vi "Log Key Value Pairs.vi"(8 "error in (no error)":errorcluster, 9 "Numeric Array Key Value Pairs":cluster{"Key":string, "Value":dbl[]}[](array[cluster]), 10 "String Key Value Pairs":cluster{"Key":string, "Value":string}[](array[cluster]), 11 "SLL Spreadsheet Logger in":refnum<class "SLL CSV Logger.lvclass">) -> (0 "error out":errorcluster, 3 "SLL Spreadsheet Logger out":refnum<class "SLL CSV Logger.lvclass">)   [LabVIEW 2014, in "SLL Spreadsheet.lvlib" / "SLL CSV Logger.lvclass"]
doc: "Provide key-value pairs to be logged, where keys will be treated as Headers.\n\nFor numeric array key-value pairs provided, each value of the array will be logged as a new row in the file. The corresponding string key-value pairs will be duplicated for each of these rows."
uses:
  SLL CSV Logger.lvclass
  SLL CSV Logger.lvclass/SLL CSV Logger.ctl
  SLL Spreadsheet.lvlib
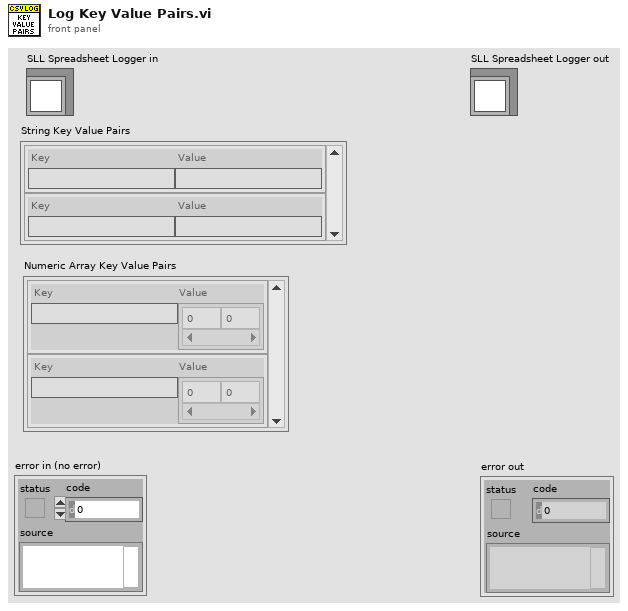
[diagram p1: front panel]
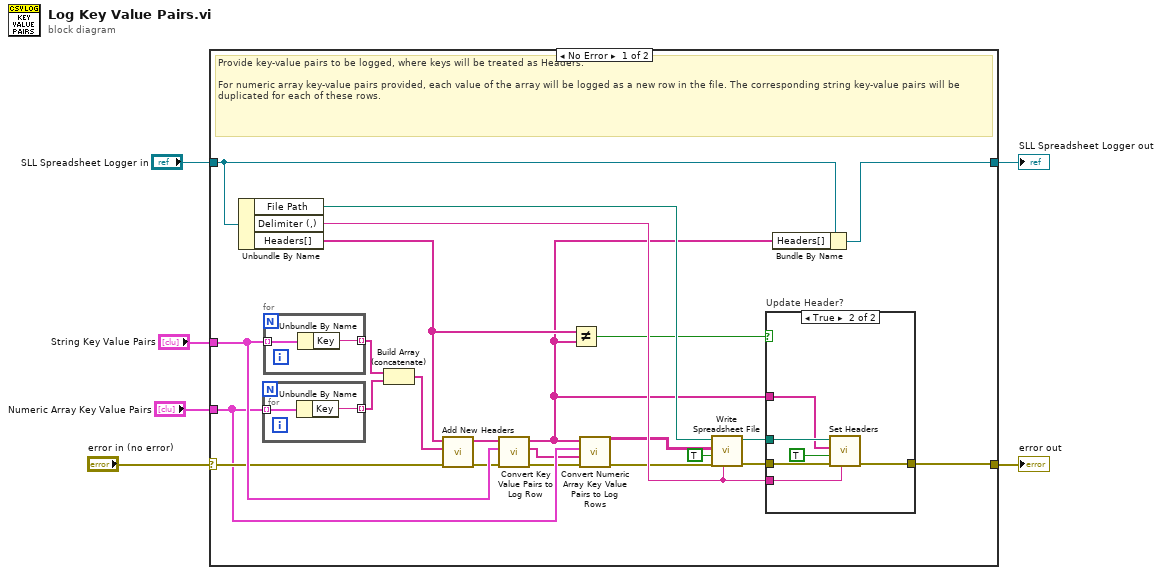
[diagram p0: block diagram]
diagram:
  n1 = case shown="No Error" "error in (no error)" {
    selector: "error in (no error)" -> [w16 w42]
    tunnel: [w21 w42] -> w5
    tunnel: [w28 w41] -> w3
    tunnel: "SLL Spreadsheet Logger in" -> [w29 w41]
    tunnel: "String Key Value Pairs" -> [w19 _]
    tunnel: "Numeric Array Key Value Pairs" -> [w11 _]
    frame No Error {
      # "Provide key-value pairs to be logged, where keys will be treated as Headers.\n\nFor numeric array key-value pairs provided, each value of the array will be logged as a new row in the file. The corresponding string key-value pairs will be duplicated for each of these rows."
      n2 = Unbundle By Name(w29) -> ("File Path"=w27:path, "Delimiter (,)"=w23:string, "Headers[]"=w20:string[])
      n3 = for {
        tunnel: w11 -> [w31] mode=indexing
        tunnel: [w30] -> w17 mode=indexing
        n4 = Unbundle By Name(w31) -> ("Key"=w30:string)
      }
      n5 = for {
        tunnel: w19 -> [w33] mode=indexing
        tunnel: [w32] -> w18 mode=indexing
        n6 = Unbundle By Name(w33) -> ("Key"=w32:string)
      }
      n7 = Build Array (concatenate)(w18, w17) -> (w15:string[])
      n8 = call "Add New Headers.vi"("error in (no error)"=w16, "Incoming Headers[]"=w15, "Existing Headers[]"=w20) -> ("error out"=w13:errorcluster, "Headers[] Out"=w14:string[])  [unwired: 7 in]
      n9 = call "Convert Key Value Pairs to Log Row.vi"("error in (no error)"=w13, "Key Value Pairs"=w19, "Headers In[]"=w14) -> ("error out"=w8:errorcluster, "Data Out[]"=w10:string[], "Headers Out[]"=w12:string[])  [unwired: 6 in]
      n10 = Not Equal?(x=w20, y=w12) -> (x != y?=w22:bool)
      n11 = call "Convert Numeric Array Key Value Pairs to Log Rows.vi"("error in (no error)"=w8, "Data[]"=w10, "Numeric Array Key Value Pairs"=w11, "Headers In[]"=w12) -> ("error out"=w7:errorcluster, "Log Data[][]"=w9:string[][])  [unwired: 6 in]
      n12 = call "Write Spreadsheet File.vi"("Delimiter (tab)"=w23, "error in (no error)"=w7, "Append to File? (F)"=TRUE, "2D String[][]"=w9, "File Path"=w27) -> ("error out"=w24:errorcluster, "File Path dup"=w25:path)  [unwired: 5 in]
      n13 = case "Update Header?" shown="True" w22 {
        tunnel: w25 -> [_ w40]
        tunnel: w24 -> [w34 w39]
        tunnel: w12 -> [_ w38]
        tunnel: w23 -> [_ w36]
        tunnel: [w34 w35] -> w21
        frame False {
        }
        frame True {
          n14 = call "Set Headers.vi"("Delimiter (,)"=w36, "error in (no error)"=w39, "Update Existing? (T)"=TRUE ("Update Existing? (F)"), "Headers[]"=w38, "File Path"=w40) -> ("error out"=w35:errorcluster)  [unwired: 5 in, 1 out]
        }
      }
      n15 = Bundle By Name(cluster=w29, "Headers[]"=w12) -> (w28:refnum<class "SLL CSV Logger.lvclass">)
    }
    frame Error {
    }
  }
  "error out" <- w5
  "SLL Spreadsheet Logger out" <- w3
